vi "GetLimits.vi"(8 "error in (no error)":errorcluster, 10 "Axis":T1 items=["1"=1, "2"=2, "3"=3, "4"=4], 11 "DelayLine in":refnum<class "DelayLine.lvclass">) -> (0 "error out":errorcluster, 1 "max":dbl, 2 "min":dbl, 3 "DelayLine out":refnum<class "DelayLine.lvclass">, 4 "real pos, mm":dbl)   [LabVIEW 2019, in "DelayLine.lvclass"]
uses:
  DelayLine.lvclass
  DelayLineLS4/LS4 axis.ctl
  DelayLine.lvclass/DelayLine.ctl
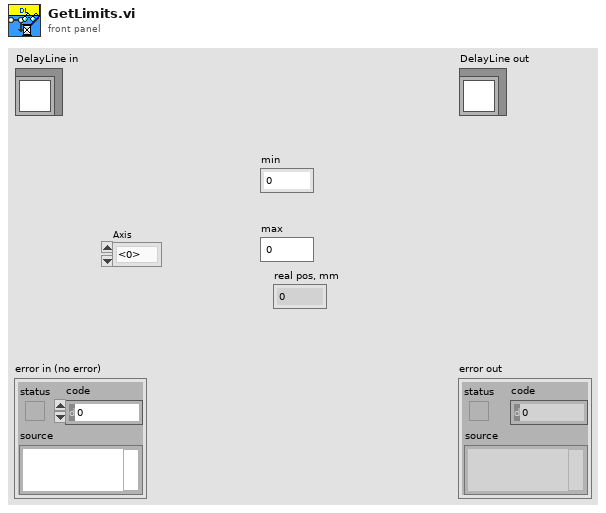
[diagram p1: front panel]
types:
  T1 = typedef "DelayLine.lvclass/LS4 axis.ctl" = u16
  T2 = cluster{"X":cluster{"Min":dbl, "Max":dbl}, "Y":cluster{"Min":dbl, "Max":dbl}, "Z":cluster{"Min":dbl, "Max":dbl}, "A":cluster{"Min":dbl, "Max":dbl}}
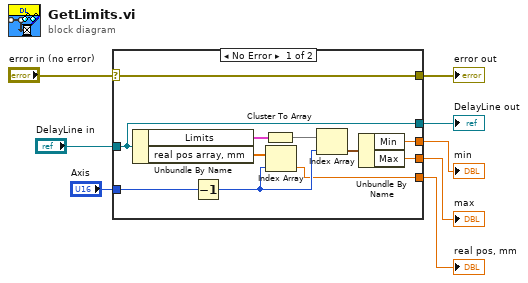
[diagram p0: block diagram]
diagram:
  n1 = case shown="No Error" "error in (no error)" {
    selector: "error in (no error)" -> [w12 w21]
    tunnel: "DelayLine in" -> [w13 w20]
    tunnel: [w13 w20] -> w3
    tunnel: [w12 w21] -> w6
    tunnel: [w15 _] -> w5
    tunnel: [w16 _] -> w4
    tunnel: "Axis" -> [w14 _]
    tunnel: [w9 _] -> w1
    frame No Error {
      n2 = Unbundle By Name(w13) -> ("Limits"=w19:T2, "real pos array, mm"=w11:dbl[])
      n3 = Decrement(x=w14) -> (x-1=w10:T1)
      n4 = Cluster To Array(cluster=w19) -> (array=w18:cluster{"Min":dbl, "Max":dbl}[])
      n5 = Index Array(array=w11, index=w10) -> (element=w9:dbl)
      n6 = Index Array(array=w18, index=w10) -> (element=w17:cluster{"Min":dbl, "Max":dbl})
      n7 = Unbundle By Name(w17) -> ("Min"=w16:dbl, "Max"=w15:dbl)
    }
    frame Error {
    }
  }
  "error out" <- w6
  "DelayLine out" <- w3
  "min" <- w4
  "max" <- w5
  "real pos, mm" <- w1
